vi "Config Measure Settings.vi"(0 "VISA resource name":refnum<visa-resource-name>, 1 "Autozero (Auto)":enum32{"Off", "Once", "Auto"}(ring)=enum."Auto", 2 "Sense (2 Wire)":enum32{"2 Wire", "4 Wire", "Calibration"}(ring), 3 "NPLC (1.000)":dbl=1.0, 5 "Node In":string, 7 "Channel (Channel A)":T1, 9 "Measure Delay (0)":dbl, 11 "error in":errorcluster, 12 "Measure Count (1)":u32=1, 13 "Interval (0.000)":dbl) -> (4 "VISA resource name out":refnum<visa-resource-name>, 6 "Node Out":string, 14 "Command String":string, 15 "error out":errorcluster)   [LabVIEW 2018, in "Keithley 2600 Series.lvlib"]
doc: "This VI configures general measurement settings that apply to all measure functions.\n\n<b>Note:</b> This VI does not configure the measurement filter. Please use Configure Measure Filter to configure the filter.\n\n<b>Functions and Attributes Used</b>\nsmuX.measure.count\nsmuX.measure.interval\nsmuX.measure.nplc"
uses:
  Keithley 2600 Series.lvlib
  Channel.ctl
  GlobalVariables.vi
panel:
  # "(c) 2008 Keithley Instruments, Inc.  ALL RIGHTS RESERVED."
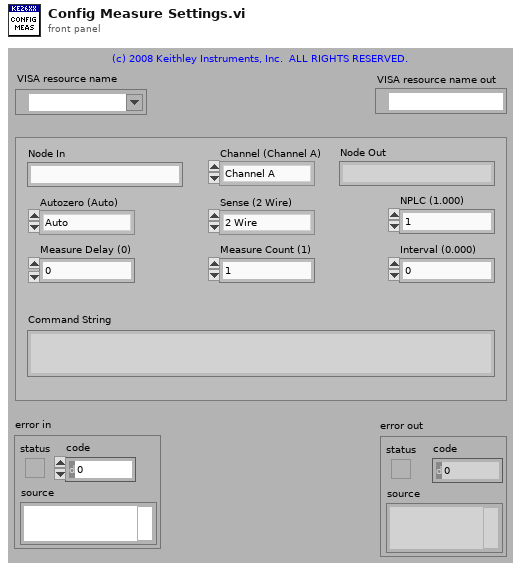
[diagram p1: front panel]
types:
  T1 = typedef "Keithley 2600 Series.lvlib/Channel.ctl" = enum32{"Channel A", "Channel B"}
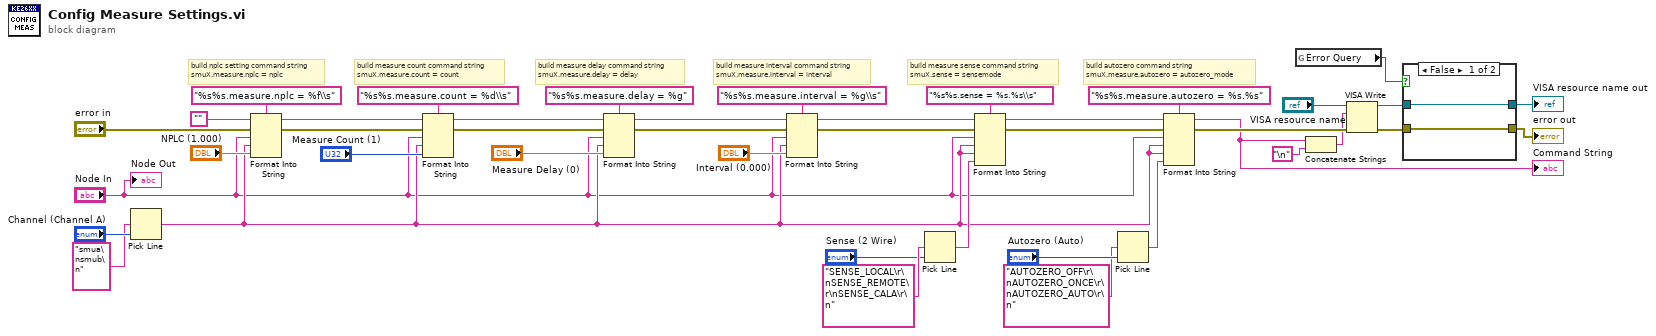
[diagram p0: block diagram]
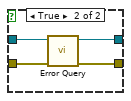
[diagram p2: hidden frame]
diagram:
  # "build measure delay command string\nsmuX.measure.delay = delay"
  # "build autozero command string\nsmuX.measure.autozero = autozero_mode"
  # "build measure sense command string\nsmuX.sense = sensemode"
  # "build measure interval command string\nsmuX.measure.interval = interval"
  # "build measure count command string\nsmuX.measure.count = count"
  # "build nplc setting command string\nsmuX.measure.nplc = nplc"
  n1 = Pick Line(multi-line string="smua\nsmub\n", line index="Channel (Channel A)") -> (output string=w5:string)  [unwired: 1 out]
  n2 = Format Into String(format string="%s%s.measure.nplc = %f\\s", initial string="", error in="error in", "Node In", w5, "NPLC (1.000)") -> (resulting string=w34:string, error out=w33:errorcluster)
  n3 = Format Into String(format string="%s%s.measure.count = %d\\s", initial string=w34, error in=w33, "Node In", w5, "Measure Count (1)") -> (resulting string=w11:string, error out=w10:errorcluster)
  n4 = Format Into String(format string="%s%s.measure.delay = %g", initial string=w11, error in=w10, "Node In", w5, "Measure Delay (0)") -> (resulting string=w8:string, error out=w9:errorcluster)
  n5 = Format Into String(format string="%s%s.measure.interval = %g\\s", initial string=w8, error in=w9, "Node In", w5, "Interval (0.000)") -> (resulting string=w18:string, error out=w17:errorcluster)
  n6 = Pick Line(multi-line string="SENSE_LOCAL\r\nSENSE_REMOTE\r\nSENSE_CALA\r\n" ("options"), line index="Sense (2 Wire)") -> (output string=w14:string)  [unwired: 1 out]
  n7 = Format Into String(format string="%s%s.sense = %s.%s\\s", initial string=w18, error in=w17, "Node In", w5, w5, w14) -> (resulting string=w16:string, error out=w15:errorcluster)
  n8 = Pick Line(multi-line string="AUTOZERO_OFF\r\nAUTOZERO_ONCE\r\nAUTOZERO_AUTO\r\n" ("options"), line index="Autozero (Auto)") -> (output string=w13:string)  [unwired: 1 out]
  n9 = Format Into String(format string="%s%s.measure.autozero = %s.%s", initial string=w16, error in=w15, "Node In", w5, w5, w13) -> (resulting string=w2:string, error out=w12:errorcluster)
  "Command String" <- w2
  n10 = global read "GlobalVariables.vi" "Error Query"() -> (w27:bool)
  n11 = Concatenate Strings(w2, "\n") -> (w1:string)
  n12 = VISA Write(VISA resource name="VISA resource name", write buffer=w1, error in (no error)=w12) -> (VISA resource name out=w29:refnum<visa-resource-name>, error out=w28:errorcluster)  [unwired: 1 out]
  n13 = case shown="False" w27 {
    tunnel: w29 -> [w44 w48]
    tunnel: w28 -> [w43 w47]
    tunnel: [w44 w46] -> w26
    tunnel: [w43 w45] -> w25
    frame False {
    }
    frame True {
      n14 = call "Error Query.vi"("error in (no error)"=w47, "VISA resource name"=w48) -> ("error out"=w45:errorcluster, "VISA resource name out"=w46:refnum<visa-resource-name>)  [unwired: 8 out]
    }
  }
  "VISA resource name out" <- w26
  "error out" <- w25
  "Node Out" <- "Node In"
